vi "Alarms Subvi.vi"(0 "H Tags":dbl[](array[numeric]), 1 "HH SP":dbl[](array[numeric]), 2 "HH Tags":dbl[](array[numeric]), 3 "Reset":bool, 5 "H SP":dbl[](array[numeric]), 9 "LTags":dbl[](array[numeric]), 11 "L SP":dbl[](array[numeric]), 12 "LL SP":dbl[](array[numeric]), 13 "LL Tage":dbl[](array[numeric])) -> (4 "HH Alarms":bool[](array[boolean]), 6 "H Alarms":bool[](array[boolean]), 10 "L Alarms":bool[](array[boolean]), 15 "LL Alarms":bool[](array[boolean]))   [LabVIEW 2013]
panel:
  out "x > y?":bool[](array[boolean])
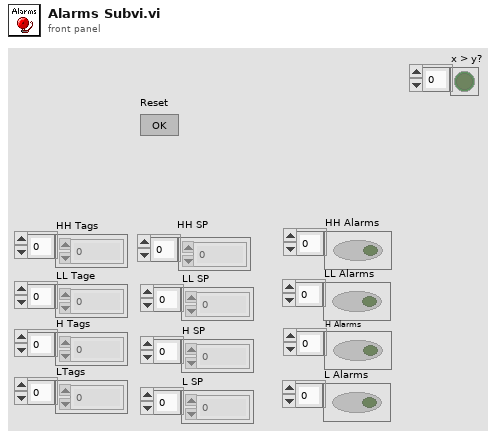
[diagram p1: front panel]
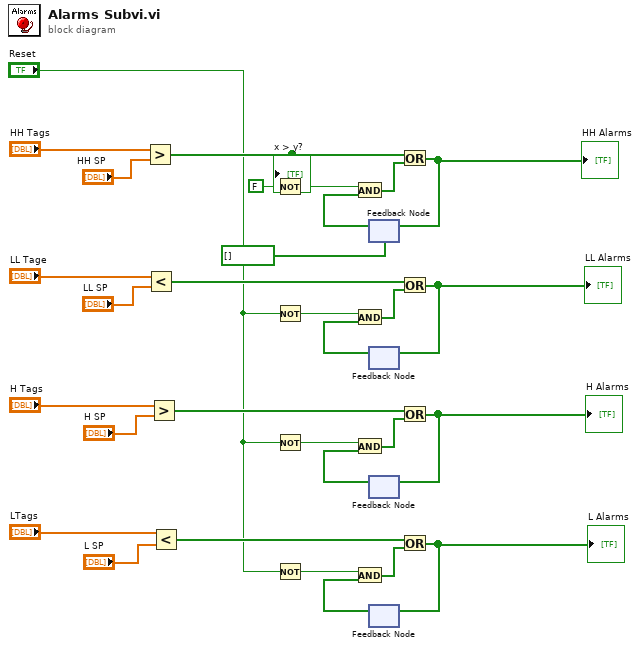
[diagram p0: block diagram]
diagram:
  n1 = Greater?(x="HH Tags", y="HH SP") -> (0:w23:bool[])
  "x > y?" <- w23
  n2 = Less?(x="LL Tage", y="LL SP") -> (x < y?=w18:bool[])
  n3 = Greater?(x="H Tags", y="H SP") -> (0:w13:bool[])
  n4 = Less?(x="LTags", y="L SP") -> (x < y?=w8:bool[])
  n5 = Not(x=FALSE) -> (.not. x?=w25:bool)
  n6 = Not(x="Reset") -> (.not. x?=w20:bool)
  n7 = Not(x="Reset") -> (.not. x?=w15:bool)
  n8 = Not(x="Reset") -> (.not. x?=w10:bool)
  n9 = feedback #1(bool[] [] ("HH Alarms 2")) -> (w26:bool[])
  n10 = And(x=w25, y=w26) -> (x .and. y?=w24:bool[])
  n11 = feedback #2() -> (w21:bool[])  [unwired: 1 in]
  n12 = And(x=w20, y=w21) -> (x .and. y?=w19:bool[])
  n13 = feedback #3() -> (w16:bool[])  [unwired: 1 in]
  n14 = And(x=w15, y=w16) -> (x .and. y?=w14:bool[])
  n15 = feedback #4() -> (w11:bool[])  [unwired: 1 in]
  n16 = And(x=w10, y=w11) -> (x .and. y?=w9:bool[])
  n17 = Or(x=w23, y=w24) -> (x .or. y?=w22:bool[])
  "HH Alarms" <- w22
  n18 = feedback-in #1(w22) -> ()
  n19 = Or(x=w18, y=w19) -> (x .or. y?=w17:bool[])
  "LL Alarms" <- w17
  n20 = feedback-in #2(w17) -> ()
  n21 = Or(x=w13, y=w14) -> (x .or. y?=w12:bool[])
  "H Alarms" <- w12
  n22 = feedback-in #3(w12) -> ()
  n23 = Or(x=w8, y=w9) -> (x .or. y?=w6:bool[])
  "L Alarms" <- w6
  n24 = feedback-in #4(w6) -> ()
